vi "Img Plot Cross.vi"(6 "Color":u32(colorbox)=6618880, 8 "error in (no error)":errorcluster, 9 "size":i32=3, 10 "position":cluster{"centerx":i32, "centery":i32}, 11 "Image In":T1) -> (0 "error out":errorcluster, 3 "Image Out":T1)   [LabVIEW 2018, in "Image Process.lvclass"]
uses:
  Image Process.lvclass
  <vilib>/vision/Image Controls.llb/IMAQ Image.ctl
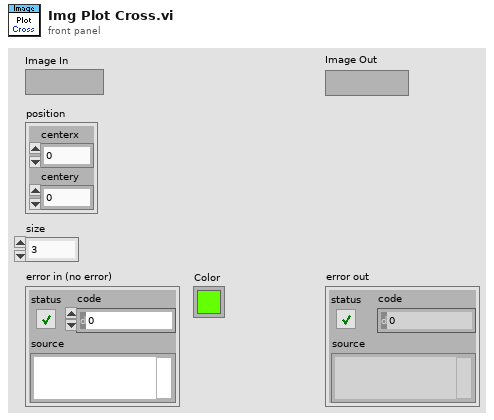
[diagram p1: front panel]
types:
  T1 = typedef "IMAQ Image.ctl" = refnum<image>
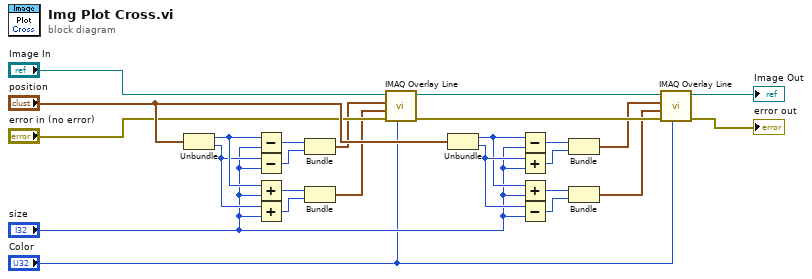
[diagram p0: block diagram]
diagram:
  n1 = Unbundle("position") -> ("centerx"=w15:i32, "centery"=w14:i32)
  n2 = Subtract(x=w15, y="size") -> (x-y=w20:i32)
  n3 = Subtract(x=w14, y="size") -> (x-y=w19:i32)
  n4 = Add(x=w15, y="size") -> (x+y=w16:i32)
  n5 = Add(x=w14, y="size") -> (x+y=w17:i32)
  n6 = Bundle(w20, w19) -> (w18:cluster{i32, i32})  [unwired: 1 in]
  n7 = Bundle(w16, w17) -> (w13:cluster{i32, i32})  [unwired: 1 in]
  n8 = call "IMAQ Overlay Line"("Color"="Color", "error in (no error)"="error in (no error)", "End Point"=w13, "Start Point"=w18, "Image"="Image In") -> ("error out"=w21:errorcluster, "Image Out"=w22:T1)  [unwired: 5 in]
  n9 = Unbundle("position") -> ("centerx"=w11:i32, "centery"=w12:i32)
  n10 = Subtract(x=w11, y="size") -> (x-y=w7:i32)
  n11 = Add(x=w12, y="size") -> (x+y=w8:i32)
  n12 = Add(x=w11, y="size") -> (x+y=w10:i32)
  n13 = Subtract(x=w12, y="size") -> (x-y=w9:i32)
  n14 = Bundle(w7, w8) -> (w5:cluster{i32, i32})  [unwired: 1 in]
  n15 = Bundle(w10, w9) -> (w4:cluster{i32, i32})  [unwired: 1 in]
  n16 = call "IMAQ Overlay Line"("Color"="Color", "error in (no error)"=w21, "End Point"=w4, "Start Point"=w5, "Image"=w22) -> ("error out"=→"error out":errorcluster, "Image Out"=→"Image Out":T1)  [unwired: 5 in]
